vi "Set MenuClass.vi"(10 "MenuClass":variant, 11 "listbox in":refnum<class "listbox.lvclass">) -> (3 "listbox out":refnum<class "listbox.lvclass">)   [LabVIEW 2016, in "listbox.lvclass"]
uses:
  listbox.lvclass
  listbox.lvclass/listbox.ctl
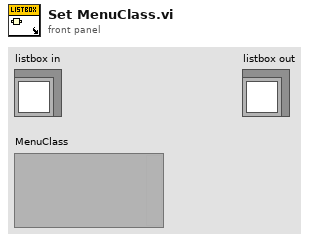
[diagram p1: front panel]
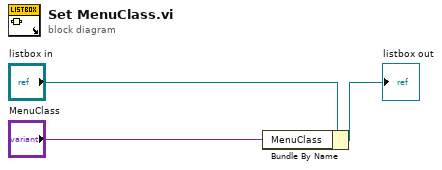
[diagram p0: block diagram]
diagram:
  n1 = Bundle By Name(cluster="listbox in", "MenuClass"="MenuClass") -> (→"listbox out":refnum<class "listbox.lvclass">)
